vi "testStatistics.vi"() -> ()   [LabVIEW 2018]
uses:
  <vilib>/measure/NI_MABase.lvlib
  277ebd99-49d9-4497-81e4-a36458fdd357.vi
  <vilib>/Analysis/NI_AALBase.lvlib
  statistics.lvlib
  statistics/StatisticsControl.ctl
panel:
  out "Numeric":i32
  out "# elements in queue 2":i32
  in  "?":enum32{"define image ", "statistics analysis"}(tab)
  out "Waveform Graph 3":dbl[](graph)
  in  "noise amplitude":dbl=0.1 format="%#.6g"
  in  "noise type":T1(ring)=enum."periodic"
  in  "amplitude":dbl=50.0 format="%#_13g"
  out "iterative":dbl[](graph)
  in  "image stat":T2=enum."image"
  out "n":i32
  out "averaged over N":dbl[][](graph)
  in  "N samples":i32=100
  in  "queue N element":i32=1 min=1
  out "# elements in queue":i32
  in  "Stop Button":bool
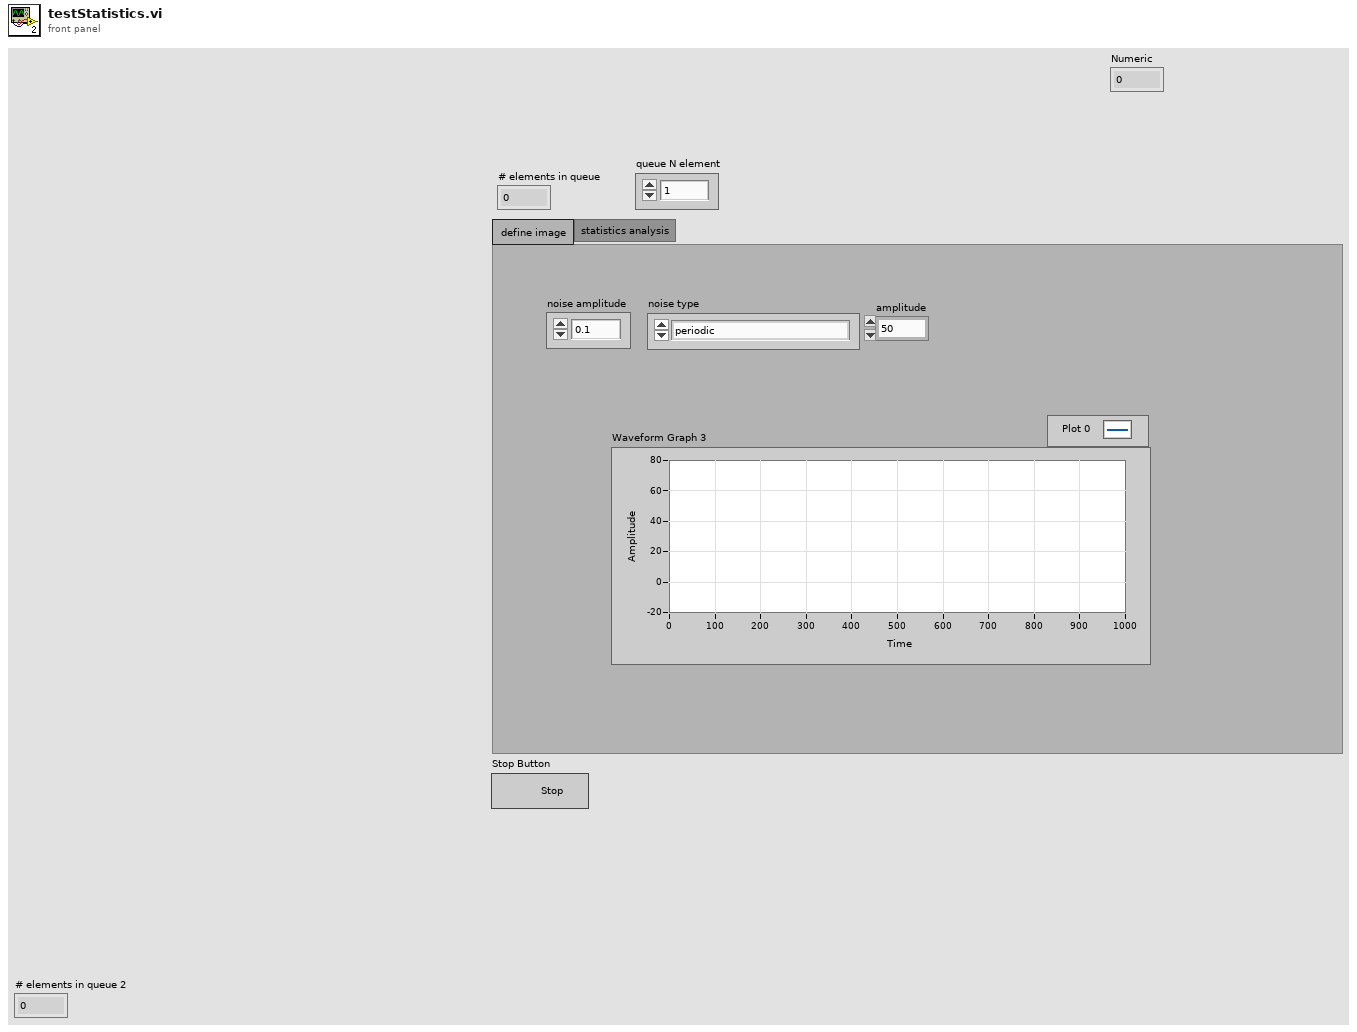
[diagram p1: front panel]
types:
  T1 = enum16{"gaussian waveform", "uniform white", "Gaussian white", "periodic", "inverse f"}
  T2 = typedef "statistics.lvlib/StatisticsControl.ctl" = enum16{"var", "image", "SNR", "std", "average"}
  T3 = cluster{"lower cutoff freq":dbl, "higher cutoff freq":dbl, "order":i32}
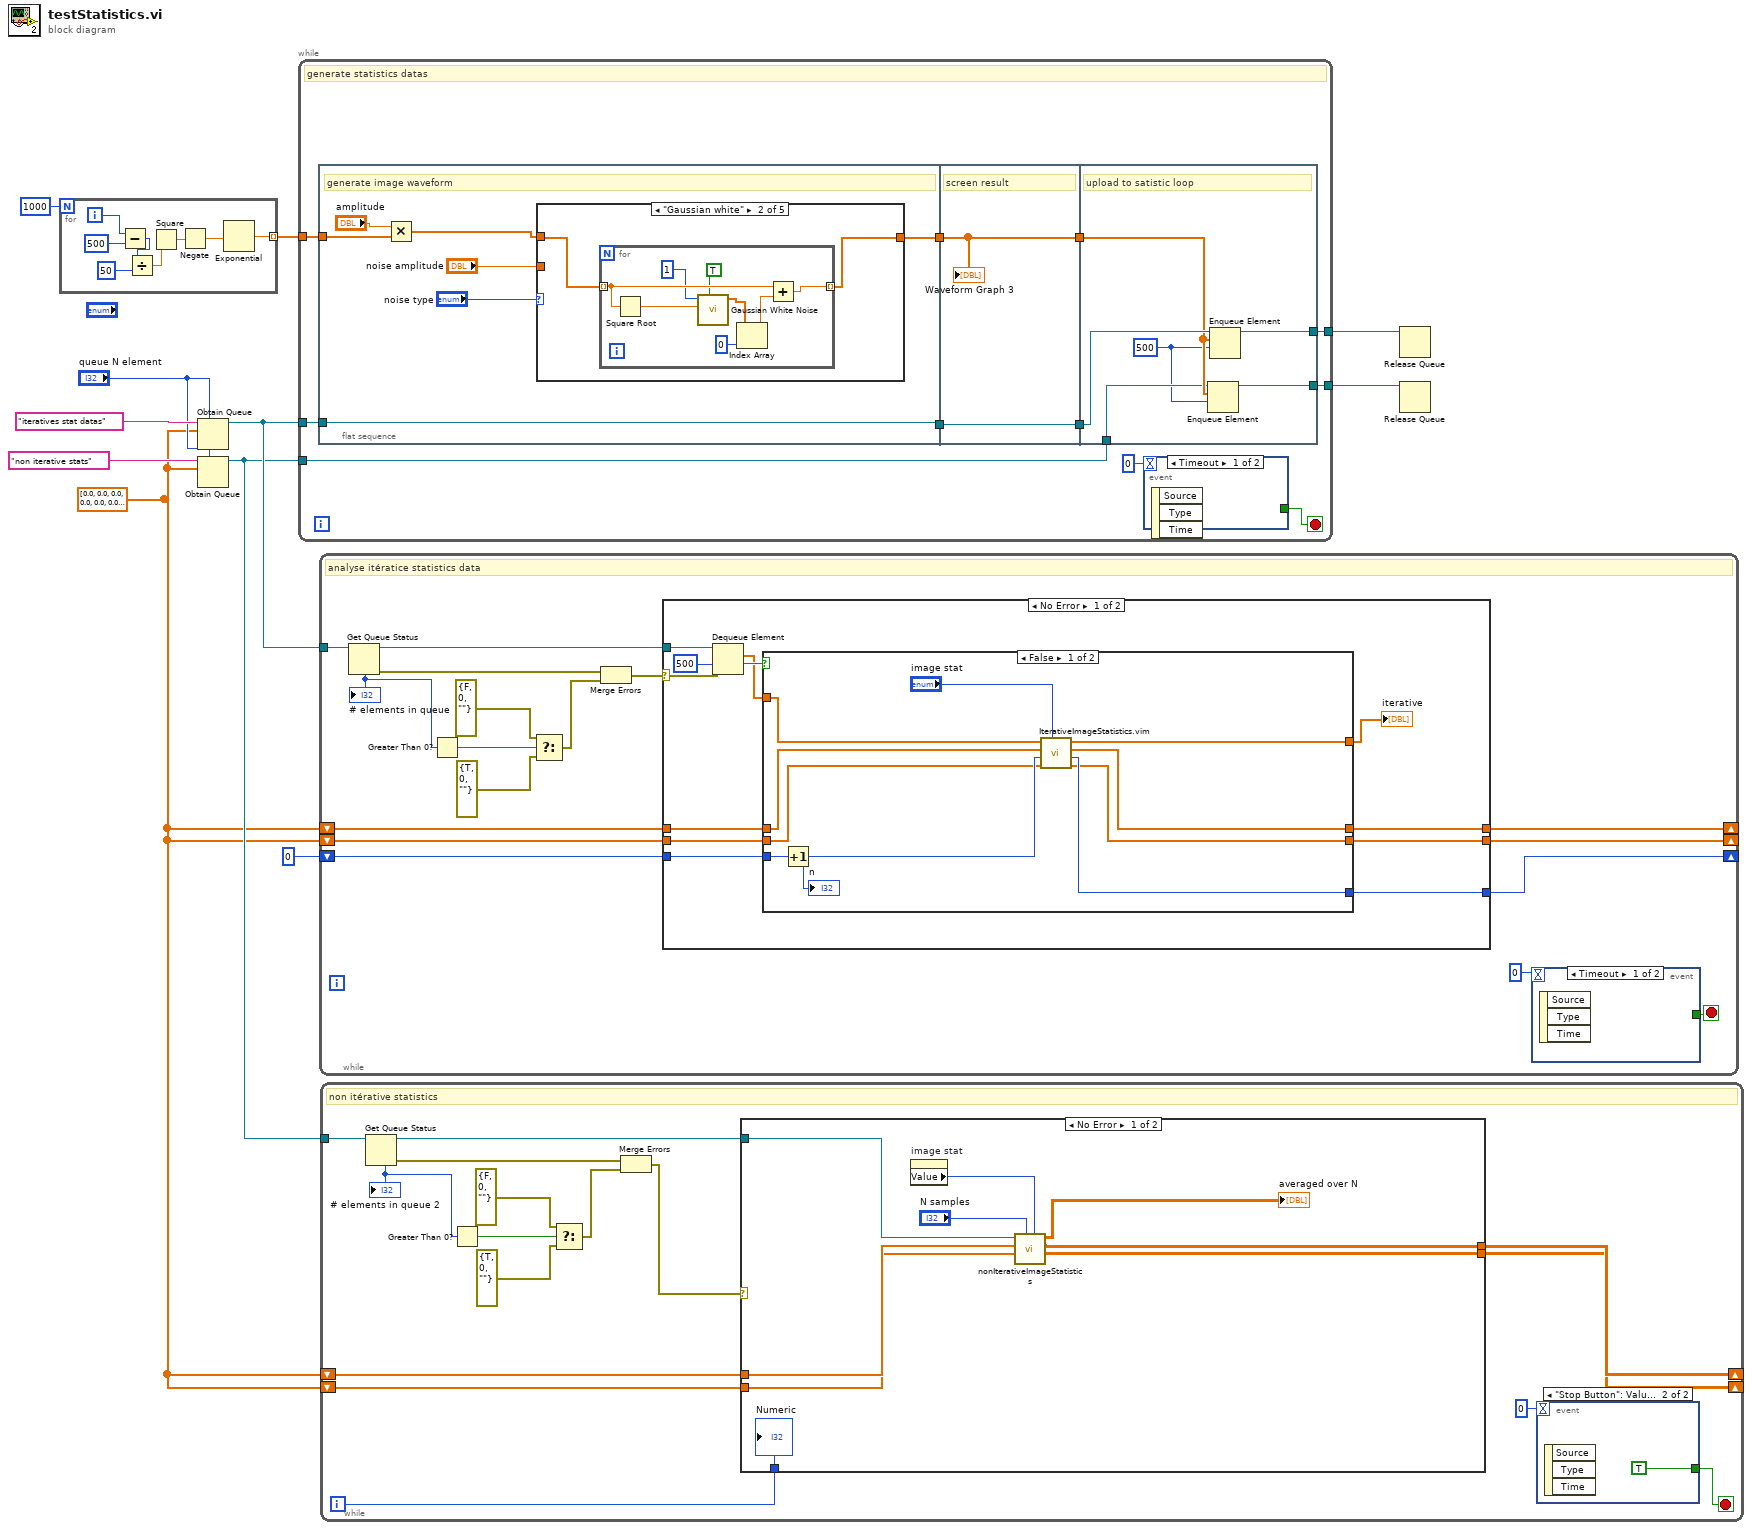
[diagram p0: block diagram]
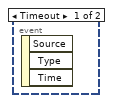
[diagram p3: hidden frame]
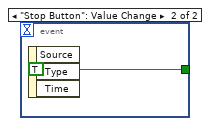
[diagram p6: hidden frame]
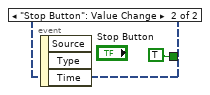
[diagram p7: hidden frame]
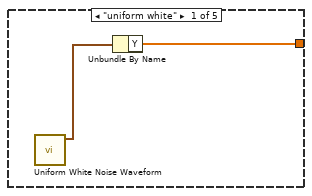
[diagram p8: hidden frame]
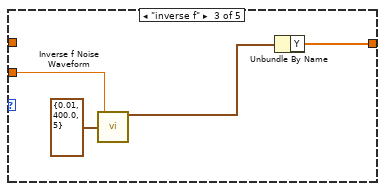
[diagram p9: hidden frame]
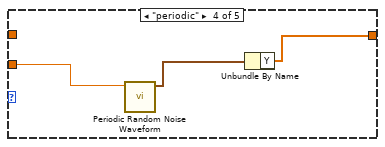
[diagram p10: hidden frame]
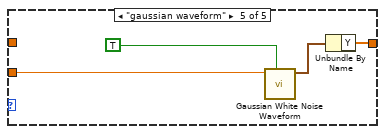
[diagram p11: hidden frame]
diagram:
  w1 = dbl[] [0.0, 0.0, 0.0, 0.0, 0.0, 0.0, 0.0, 0.0, 0.0, 0.0, 0.0, 0.0, 0.0, 0.0, 0.0, 0.0, 0.0, 0.0, 0.0, 0.0, 0.0, 0.0, 0.0, 0.0, 0.0, 0.0, 0.0, 0.0, 0.0, 0.0, 0.0, 0.0, 0.0, 0.0, 0.0, 0.0, 0.0, 0.0, 0.0, 0.0, 0.0, 0.0, 0.0, 0.0, 0.0, 0.0, 0.0, 0.0, 0.0, 0.0, 0.0, 0.0, 0.0, 0.0, 0.0, 0.0, 0.0, 0.0, 0.0, 0.0, 0.0, 0.0, 0.0, 0.0, 0.0, 0.0, 0.0, 0.0, 0.0, 0.0, 0.0, 0.0, 0.0, 0.0, 0.0, 0.0, 0.0, 0.0, 0.0, 0.0, 0.0, 0.0, 0.0, 0.0, 0.0, 0.0, 0.0, 0.0, 0.0, 0.0, 0.0, 0.0, 0.0, 0.0, 0.0, 0.0, 0.0, 0.0, 0.0, 0.0, 0.0, 0.0, 0.0, 0.0, 0.0, 0.0, 0.0, 0.0, 0.0, 0.0, 0.0, 0.0, 0.0, 0.0, 0.0, 0.0, 0.0, 0.0, 0.0, 0.0, 0.0, 0.0, 0.0, 0.0, 0.0, 0.0, 0.0, 0.0, 0.0, 0.0, 0.0, 0.0, 0.0, 0.0, 0.0, 0.0, 0.0, 0.0, 0.0, 0.0, 0.0, 0.0, 0.0, 0.0, 0.0, 0.0, 0.0, 0.0, 0.0, 0.0, 0.0, 0.0, 0.0, 0.0, 0.0, 0.0, 0.0, 0.0, 0.0, 0.0, 0.0, 0.0, 0.0, 0.0, 0.0, 0.0, 0.0, 0.0, 0.0, 0.0, 0.0, 0.0, 0.0, 0.0, 0.0, 0.0, 0.0, 0.0, 0.0, 0.0, 0.0, 0.0, 0.0, 0.0, 0.0, 0.0, 0.0, 0.0, 0.0, 0.0, 0.0, 0.0, 0.0, 0.0, 0.0, 0.0, 0.0, 0.0, 0.0, 0.0, 0.0, 0.0, 0.0, 0.0, 0.0, 0.0, 0.0, 0.0, 0.0, 0.0, 0.0, 0.0, 0.0, 0.0, 0.0, 0.0, 0.0, 0.0, 0.0, 0.0, 0.0, 0.0, 0.0, 0.0, 0.0, 0.0, 0.0, 0.0, 0.0, 0.0, 0.0, 0.0, 0.0, 0.0, 0.0, 0.0, 0.0, 0.0, 0.0, 0.0, 0.0, 0.0, 0.0, 0.0, 0.0, 0.0, 0.0, 0.0, 0.0, 0.0, 0.0, 0.0, 0.0, 0.0, 0.0, 0.0, 0.0, 0.0, 0.0, 0.0, 0.0, 0.0, 0.0, 0.0, 0.0, 0.0, 0.0, 0.0, 0.0, 0.0, 0.0, 0.0, 0.0, 0.0, 0.0, 0.0, 0.0, 0.0, 0.0, 0.0, 0.0, 0.0, 0.0, 0.0, 0.0, 0.0, 0.0, 0.0, 0.0, 0.0, 0.0, 0.0, 0.0, 0.0, 0.0, 0.0, 0.0, 0.0, 0.0, 0.0, 0.0, 0.0, 0.0, 0.0, 0.0, 0.0, 0.0, 0.0, 0.0, 0.0, 0.0, 0.0, 0.0, 0.0, 0.0, 0.0, 0.0, 0.0, 0.0, 0.0, 0.0, 0.0, 0.0, 0.0, 0.0, 0.0, 0.0, 0.0, 0.0, 0.0, 0.0, 0.0, 0.0, 0.0, 0.0, 0.0, 0.0, 0.0, 0.0, 0.0, 0.0, 0.0, 0.0, 0.0, 0.0, 0.0, 0.0, 0.0, 0.0, 0.0, 0.0, 0.0, 0.0, 0.0, 0.0, 0.0, 0.0, 0.0, 0.0, 0.0, 0.0, 0.0, 0.0, 0.0, 0.0, 0.0, 0.0, 0.0, 0.0, 0.0, 0.0, 0.0, 0.0, 0.0, 0.0, 0.0, 0.0, 0.0, 0.0, 0.0, 0.0, 0.0, 0.0, 0.0, 0.0, 0.0, 0.0, 0.0, 0.0, 0.0, 0.0, 0.0, 0.0, 0.0, 0.0, 0.0, 0.0, 0.0, 0.0, 0.0, 0.0, 0.0, 0.0, 0.0, 0.0, 0.0, 0.0, 0.0, 0.0, 0.0, 0.0, 0.0, 0.0, 0.0, 0.0, 0.0, 0.0, 0.0, 0.0, 0.0, 0.0, 0.0, 0.0, 0.0, 0.0, 0.0, 0.0, 0.0, 0.0, 0.0, 0.0, 0.0, 0.0, 0.0, 0.0, 0.0, 0.0, 0.0, 0.0, 0.0, 0.0, 0.0, 0.0, 0.0, 0.0, 0.0, 0.0, 0.0, 0.0, 0.0, 0.0, 0.0, 0.0, 0.0, 0.0, 0.0, 0.0, 0.0, 0.0, 0.0, 0.0, 0.0, 0.0, 0.0, 0.0, 0.0, 0.0, 0.0, 0.0, 0.0, 0.0, 0.0, 0.0, 0.0, 0.0, 0.0, 0.0, 0.0, 0.0, 0.0, 0.0, 0.0, 0.0, 0.0, 0.0, 0.0, 0.0, 0.0, 0.0, 0.0, 0.0, 0.0, 0.0, 0.0, 0.0, 0.0, 0.0, 0.0, 0.0, 0.0, 0.0, 0.0, 0.0, 0.0, 0.0, 0.0, 0.0, 0.0, 0.0, 0.0, 0.0, 0.0, 0.0, 0.0, 0.0, 0.0, 0.0, 0.0, 0.0, 0.0, 0.0, 0.0, 0.0, 0.0, 0.0, 0.0, 0.0, 0.0, 0.0, 0.0, 0.0, 0.0, 0.0, 0.0, 0.0, 0.0, 0.0, 0.0, 0.0, 0.0, 0.0, 0.0, 0.0, 0.0, 0.0, 0.0, 0.0, 0.0, 0.0, 0.0, 0.0, 0.0, 0.0, 0.0, 0.0, 0.0, 0.0, 0.0, 0.0, 0.0, 0.0, 0.0, 0.0, 0.0, 0.0, 0.0, 0.0, 0.0, 0.0, 0.0, 0.0, 0.0, 0.0, 0.0, 0.0, 0.0, 0.0, 0.0, 0.0, 0.0, 0.0, 0.0, 0.0, 0.0, 0.0, 0.0, 0.0, 0.0, 0.0, 0.0, 0.0, 0.0, 0.0, 0.0, 0.0, 0.0, 0.0, 0.0, 0.0, 0.0, 0.0, 0.0, 0.0, 0.0, 0.0, 0.0, 0.0, 0.0, 0.0, 0.0, 0.0, 0.0, 0.0, 0.0, 0.0, 0.0, 0.0, 0.0, 0.0, 0.0, 0.0, 0.0, 0.0, 0.0, 0.0, 0.0, 0.0, 0.0, 0.0, 0.0, 0.0, 0.0, 0.0, 0.0, 0.0, 0.0, 0.0, 0.0, 0.0, 0.0, 0.0, 0.0, 0.0, 0.0, 0.0, 0.0, 0.0, 0.0, 0.0, 0.0, 0.0, 0.0, 0.0, 0.0, 0.0, 0.0, 0.0, 0.0, 0.0, 0.0, 0.0, 0.0, 0.0, 0.0, 0.0, 0.0, 0.0, 0.0, 0.0, 0.0, 0.0, 0.0, 0.0, 0.0, 0.0, 0.0, 0.0, 0.0, 0.0, 0.0, 0.0, 0.0, 0.0, 0.0, 0.0, 0.0, 0.0, 0.0, 0.0, 0.0, 0.0, 0.0, 0.0, 0.0, 0.0, 0.0, 0.0, 0.0, 0.0, 0.0, 0.0, 0.0, 0.0, 0.0, 0.0, 0.0, 0.0, 0.0, 0.0, 0.0, 0.0, 0.0, 0.0, 0.0, 0.0, 0.0, 0.0, 0.0, 0.0, 0.0, 0.0, 0.0, 0.0, 0.0, 0.0, 0.0, 0.0, 0.0, 0.0, 0.0, 0.0, 0.0, 0.0, 0.0, 0.0, 0.0, 0.0, 0.0, 0.0, 0.0, 0.0, 0.0, 0.0, 0.0, 0.0, 0.0, 0.0, 0.0, 0.0, 0.0, 0.0, 0.0, 0.0, 0.0, 0.0, 0.0, 0.0, 0.0, 0.0, 0.0, 0.0, 0.0, 0.0, 0.0, 0.0, 0.0, 0.0, 0.0, 0.0, 0.0, 0.0, 0.0, 0.0, 0.0, 0.0, 0.0, 0.0, 0.0, 0.0, 0.0, 0.0, 0.0, 0.0, 0.0, 0.0, 0.0, 0.0, 0.0, 0.0, 0.0, 0.0, 0.0, 0.0, 0.0, 0.0, 0.0, 0.0, 0.0, 0.0, 0.0, 0.0, 0.0, 0.0, 0.0, 0.0, 0.0, 0.0, 0.0, 0.0, 0.0, 0.0, 0.0, 0.0, 0.0, 0.0, 0.0, 0.0, 0.0, 0.0, 0.0, 0.0, 0.0, 0.0, 0.0, 0.0, 0.0, 0.0, 0.0, 0.0, 0.0, 0.0, 0.0, 0.0, 0.0, 0.0, 0.0, 0.0, 0.0, 0.0, 0.0, 0.0, 0.0, 0.0, 0.0, 0.0, 0.0, 0.0, 0.0, 0.0, 0.0, 0.0, 0.0, 0.0, 0.0, 0.0, 0.0, 0.0, 0.0, 0.0, 0.0, 0.0, 0.0, 0.0, 0.0, 0.0, 0.0, 0.0, 0.0, 0.0, 0.0, 0.0, 0.0, 0.0, 0.0, 0.0, 0.0, 0.0, 0.0, 0.0, 0.0, 0.0, 0.0, 0.0, 0.0, 0.0, 0.0, 0.0, 0.0, 0.0, 0.0, 0.0, 0.0, 0.0, 0.0, 0.0, 0.0, 0.0, 0.0, 0.0, 0.0, 0.0, 0.0, 0.0, 0.0, 0.0, 0.0, 0.0, 0.0, 0.0, 0.0, 0.0, 0.0, 0.0, 0.0, 0.0, 0.0, 0.0, 0.0, 0.0, 0.0, 0.0, 0.0, 0.0, 0.0, 0.0, 0.0, 0.0, 0.0, 0.0, 0.0, 0.0, 0.0, 0.0, 0.0, 0.0, 0.0, 0.0, 0.0, 0.0, 0.0, 0.0, 0.0, 0.0, 0.0, 0.0, 0.0, 0.0, 0.0, 0.0, 0.0, 0.0, 0.0, 0.0, 0.0, 0.0, 0.0, 0.0, 0.0, 0.0, 0.0, 0.0, 0.0, 0.0, 0.0, 0.0, 0.0, 0.0, 0.0, 0.0, 0.0, 0.0, 0.0, 0.0, 0.0, 0.0, 0.0, 0.0, 0.0, 0.0, 0.0, 0.0, 0.0, 0.0, 0.0, 0.0, 0.0, 0.0, 0.0, 0.0, 0.0, 0.0, 0.0, 0.0, 0.0, 0.0, 0.0, 0.0, 0.0, 0.0, 0.0] ("Y")
  n1 = for {
    N: 1000 -> [_]
    tunnel: [w15] -> w6 mode=indexing
    i -> [w19]
    n2 = Subtract(x=w19, y=500) -> (x-y=w14:i32)
    n3 = Divide(x=w14, y=50) -> (x/y=w12:dbl)
    n4 = Square(x=w12) -> (x^2=w17:dbl)
    n5 = Negate(x=w17) -> (-x=w16:dbl)
    n6 = Exponential(1:w16) -> (0:w15:dbl)
  }
  n7 = Obtain Queue(max queue size (-1, unlimited)="queue N element", name (unnamed)="iteratives stat datas", element data type=w1) -> (queue out=w11:refnum<queue>)  [unwired: 2 in, 2 out]
  n8 = Obtain Queue(max queue size (-1, unlimited)="queue N element", name (unnamed)="non iterative stats", element data type=w1) -> (queue out=w2:refnum<queue>)  [unwired: 2 in, 2 out]
  n9 = while {
    tunnel: w11 -> [w27]
    tunnel: [w24] -> w9
    tunnel: w6 -> [w22]
    tunnel: w2 -> [w21]
    tunnel: [w20] -> w3
    stop <- w29 stop-if-true
    # "generate statistics datas"
    n10 = flat-sequence {
      tunnel: [w35] -> w30
      tunnel: w27 -> [w36]
      tunnel: [w36] -> w26
      tunnel: w22 -> [w34]
      tunnel: w30 -> [w62]
      tunnel: w26 -> [w63]
      tunnel: [w63] -> w25
      tunnel: [w62] -> w23
      tunnel: w25 -> [w69]
      tunnel: [w68] -> w24
      tunnel: w23 -> [w67]
      tunnel: w21 -> [w66]
      tunnel: [w64] -> w20
      frame #0 {
        # "generate image waveform"
        n11 = Multiply(x="amplitude", y=w34) -> (x*y=w33:dbl[])
        n12 = case shown="\"Gaussian white\"" "noise type" {
          tunnel: "noise amplitude" -> [_ _ w53 w57 w60]
          tunnel: [w39 w41 w51 w55 w58] -> w35
          tunnel: w33 -> [_ w42 _ _ _]
          frame "uniform white" {
            n13 = call <vilib>:"Uniform White Noise Waveform.vi"() -> ("signal out"=w40:waveform(dbl))  [unwired: 10 in, 1 out]
            n14 = Unbundle By Name(w40) -> ("Y"=w39:dbl[])
          }
          frame "Gaussian white" {
            n15 = for {
              tunnel: w42 -> [w50] mode=indexing
              tunnel: [w48] -> w41 mode=indexing
              n16 = Square Root(x=w50) -> (sqrt(x)=w43:dbl)
              n17 = call <vilib>:"Gaussian White Noise.vi"("initialize?"=TRUE, "standard deviation"=w43, "samples"=1) -> ("Gaussian noise pattern"=w47:dbl[])  [unwired: 7 in, 1 out]
              n18 = Index Array(array=w47, index=0) -> (element=w45:dbl)
              n19 = Add(x=w50, y=w45) -> (x+y=w48:dbl)
            }
          }
          frame "inverse f" {
            n20 = call <vilib>:"Inverse f Noise Waveform.vi"("noise density"=w53, "filter specifications"=T3 {"lower cutoff freq"=0.01, "higher cutoff freq"=400.0, "order"=5}) -> ("signal out"=w52:waveform(dbl))  [unwired: 9 in, 4 out]
            n21 = Unbundle By Name(w52) -> ("Y"=w51:dbl[])
          }
          frame "periodic" {
            n22 = call <vilib>:"Periodic Random Noise Waveform.vi"("spectral amplitude"=w57) -> ("signal out"=w56:waveform(dbl))  [unwired: 9 in, 1 out]
            n23 = Unbundle By Name(w56) -> ("Y"=w55:dbl[])
          }
          frame "gaussian waveform" {
            n24 = call <vilib>:"Gaussian White Noise Waveform.vi"("reset signal"=TRUE, "standard deviation"=w60) -> ("signal out"=w61:waveform(dbl))  [unwired: 8 in, 1 out]
            n25 = Unbundle By Name(w61) -> ("Y"=w58:dbl[])
          }
        }
      }
      frame #1 {
        # "screen result"
        "Waveform Graph 3" <- w62
      }
      frame #2 {
        w65 = 500 ("timeout in ms (-1)")
        # "upload to satistic loop"
        n26 = Enqueue Element(queue=w66, element=w67, timeout in ms (-1)=w65) -> (queue out=w64:refnum<queue>)  [unwired: 1 in, 2 out]
        n27 = Enqueue Element(queue=w69, element=w67, timeout in ms (-1)=w65) -> (queue out=w68:refnum<queue>)  [unwired: 1 in, 2 out]
      }
    }
    n28 = event shown="[0] Timeout" {
      selector: _ -> [_ _]
      dyn-events: _ -> [_ _]
      timeout: 0 -> [_ _]
      tunnel: [_ TRUE] -> w29
      event Timeout {
        n29 = event-data() -> ()  [unwired: 1 in, 3 out]
      }
      event "Stop Button": Value Change {
        n30 = event-data() -> ()  [unwired: 1 in, 3 out]
      }
    }
  }
  n31 = while {
    tunnel: w11 -> [w85]
    shift-right: [w71] -> _
    shift-left: w1 -> [w83]
    shift-right: [w81] -> _
    shift-left: 0 -> [w82]
    shift-right: [w70] -> _
    shift-left: w1 -> [w72]
    stop <- w86 stop-if-true
    # "analyse itératice statistics data"
    n32 = Get Queue Status(queue=w85) -> (queue out=w84:refnum<queue>, error out=w75:errorcluster, # elements in queue=w73:i32)  [unwired: 2 in, 5 out]
    "# elements in queue" <- w73
    n33 = Greater Than 0?(x=w73) -> (x > 0?=w79:bool)
    n34 = Select(t=errorcluster {"status"=FALSE, "code"=0, "source"=""} ("error constant"), s=w79, f=errorcluster {"status"=TRUE, "code"=0, "source"=""} ("error constant")) -> (s? t:f=w76:errorcluster)
    n35 = Merge Errors(w75, w76) -> (w74:errorcluster)
    n36 = case shown="No Error" w74 {
      selector: w74 -> [w98 _]
      tunnel: w84 -> [w97 _]
      tunnel: w83 -> [w93 w114]
      tunnel: w82 -> [w92 w115]
      tunnel: [w91 w115] -> w81
      tunnel: [w90 w114] -> w71
      tunnel: [w89 w113] -> w70
      tunnel: w72 -> [w88 w113]
      frame No Error {
        n37 = Dequeue Element(queue=w97, timeout in ms (-1)=500, error in (no error)=w98) -> (element=w94:dbl[], timed out?=w95:bool)  [unwired: 2 out]
        n38 = case shown="False" w95 {
          tunnel: w94 -> [w101 w109]
          tunnel: [w107 w109] -> w87
          tunnel: w93 -> [w100 w111]
          tunnel: w92 -> [w108 w112]
          tunnel: [w105 w112] -> w91
          tunnel: [w103 w111] -> w90
          tunnel: [w102 w110] -> w89
          tunnel: w88 -> [w99 w110]
          frame False {
            n39 = Increment(x=w108) -> (x+1=w106:i32)
            "n" <- w106
            n40 = call "IterativeImageStatistics.vim"("image stat"="image stat", "Var n"=w99, "iterative index"=w106, "Mu n"=w100, "image n"=w101) -> ("Var n+1"=w102:dbl[], "iterative index out"=w105:i32, "MU n+1"=w103:dbl[], "stat OUT"=w107:dbl[])  [unwired: 3 in]
          }
          frame True {
          }
        }
        "iterative" <- w87
      }
      frame Error {
      }
    }
    n41 = event shown="[0] Timeout" {
      selector: _ -> [_ _]
      dyn-events: _ -> [_ _]
      timeout: 0 -> [_ _]
      tunnel: [_ TRUE] -> w86
      event Timeout {
        n42 = event-data() -> ()  [unwired: 1 in, 3 out]
      }
      event "Stop Button": Value Change {
        n43 = event-data() -> ()  [unwired: 1 in, 3 out]
      }
    }
  }
  n44 = while {
    tunnel: w2 -> [w124]
    shift-right: [w121] -> _
    shift-left: w1 -> [w119]
    shift-right: [w120] -> _
    shift-left: w1 -> [w118]
    i -> [w117]
    stop <- w131 stop-if-true
    # "non itérative statistics"
    n45 = Get Queue Status(queue=w124) -> (queue out=w122:refnum<queue>, error out=w126:errorcluster, # elements in queue=w125:i32)  [unwired: 2 in, 5 out]
    "# elements in queue 2" <- w125
    n46 = Greater Than 0?(x=w125) -> (x > 0?=w130:bool)
    n47 = Select(t=errorcluster {"status"=FALSE, "code"=0, "source"=""} ("error constant"), s=w130, f=errorcluster {"status"=TRUE, "code"=0, "source"=""} ("error constant")) -> (s? t:f=w127:errorcluster)
    n48 = Merge Errors(w126, w127) -> (w123:errorcluster)
    n49 = case shown="No Error" w123 {
      tunnel: w122 -> [w141 _]
      tunnel: [w139 w143] -> w121
      tunnel: [w138 w142] -> w120
      tunnel: w119 -> [w137 w142]
      tunnel: w118 -> [w136 w143]
      tunnel: w117 -> [w134 _]
      frame No Error {
        n50 = property on="image stat" class="Enum (strict)"() -> ("Value"=w140:T2)  [unwired: 2 in, 2 out]
        n51 = call "nonIterativeImageStatistics.vi"("image stat"=w140, "N samples"="N samples", "var n"=w136, "MU n"=w137, "elements in"=w141) -> ("var n+1"=w138:dbl[][], "MU n+1"=w139:dbl[][], "stat out"=→"averaged over N":dbl[][])  [unwired: 4 in]
        "Numeric" <- w134
      }
      frame Error {
      }
    }
    n52 = event shown="[1] \"Stop Button\": Value Change" {
      selector: _ -> [_ _]
      dyn-events: _ -> [_ _]
      timeout: 0 -> [_ _]
      tunnel: [_ TRUE] -> w131
      event Timeout {
        n53 = event-data() -> ()  [unwired: 1 in, 3 out]
      }
      event "Stop Button": Value Change {
        n54 = event-data() -> ()  [unwired: 1 in, 3 out]
      }
    }
  }
  n55 = Release Queue(queue=w9) -> ()  [unwired: 2 in, 3 out]
  n56 = Release Queue(queue=w3) -> ()  [unwired: 2 in, 3 out]
